vi "Read Servo Switch.vi"(8 "error in (no error)":errorcluster, 11 "tCRD in":refnum<class "Open Path CRD.lvclass">) -> (0 "error out":errorcluster, 2 "Servo Switch":refnum<class "Servo Switch.lvclass">, 3 "tCRD out":refnum<class "Open Path CRD.lvclass">)   [LabVIEW 2015, in "Open Path CRD.lvclass"]
uses:
  Open Path CRD.lvclass
  Switch/Servo Switch.lvclass
  Open Path CRD.lvclass/Open Path CRD.ctl
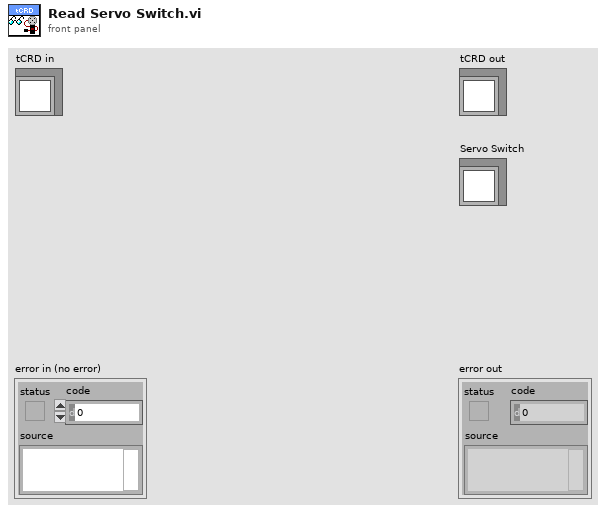
[diagram p1: front panel]
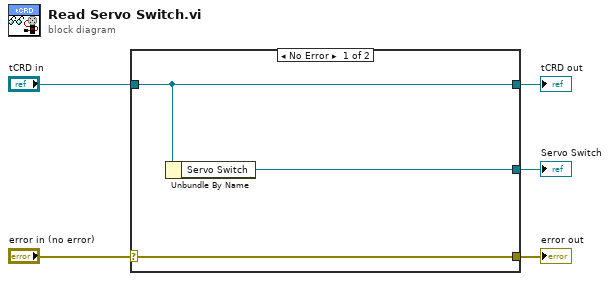
[diagram p0: block diagram]
diagram:
  n1 = case shown="No Error" "error in (no error)" {
    selector: "error in (no error)" -> [w8 w9]
    tunnel: [w8 w9] -> w4
    tunnel: [w7 w10] -> w2
    tunnel: "tCRD in" -> [w7 w10]
    tunnel: [w6 _] -> w1
    frame No Error {
      n2 = Unbundle By Name(w7) -> ("Servo Switch"=w6:refnum<class "Servo Switch.lvclass">)
    }
    frame Error {
    }
  }
  "error out" <- w4
  "tCRD out" <- w2
  "Servo Switch" <- w1
